vi "CAN Log Queue FGV Create the Reference.vi"(8 "error in":errorcluster, 11 "Selected Sockets":i16[](array[numeric])) -> (0 "error out":errorcluster)   [LabVIEW 2023, in "LTT_TeststandSteptypes.lvlib"]
uses:
  LTT_TeststandSteptypes.lvlib
  Control/CAN FGV State.ctl
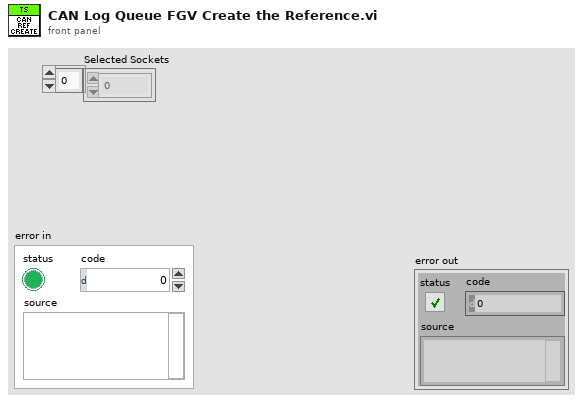
[diagram p1: front panel]
types:
  T1 = typedef "LTT_TeststandSteptypes.lvlib/CAN FGV State.ctl" = enum16{"Init", "Get", "Set"}
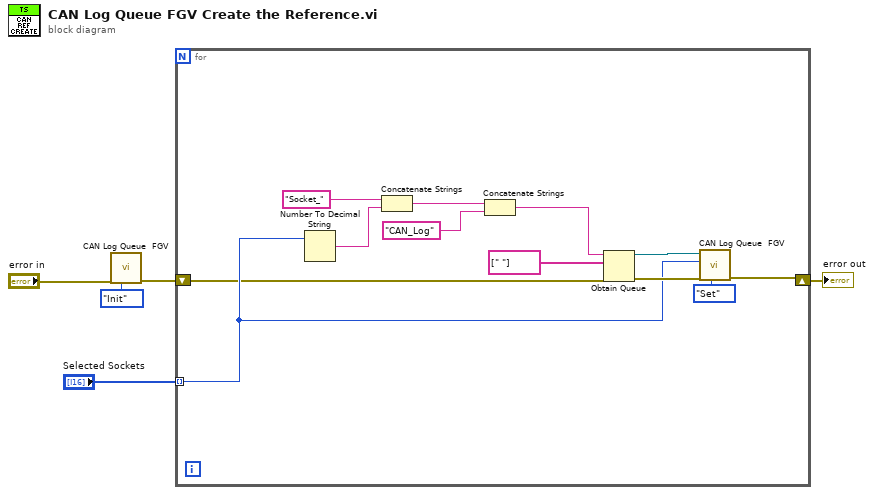
[diagram p0: block diagram]
diagram:
  n1 = call "CAN Log Queue  FGV.vi"("CAN FGV State"=CAN_FGV_State."Init", "error in"="error in") -> ("error out"=w2:errorcluster)  [unwired: 8 in, 1 out]
  n2 = for {
    tunnel: "Selected Sockets" -> [w7] mode=indexing
    shift-right: [w8] -> w1
    shift-left: w2 -> [w6]
    n3 = Number To Decimal String(number=w7) -> (decimal integer string=w16:string)  [unwired: 1 in]
    n4 = Concatenate Strings("Socket_" ("name (unnamed)"), w16) -> (w15:string)
    n5 = Concatenate Strings(w15, "CAN_Log" ("string")) -> (w14:string)
    n6 = Obtain Queue(name (unnamed)=w14, element data type=string[] [" "] ("appended array"), error in (no error)=w6) -> (queue out=w11:refnum<queue>, error out=w10:errorcluster)  [unwired: 2 in, 1 out]
    n7 = call "CAN Log Queue  FGV.vi"("CAN FGV State"=CAN_FGV_State."Set", "error in"=w10, "Current Scoket"=w7, "Log queue in"=w11) -> ("error out"=w8:errorcluster)  [unwired: 6 in, 1 out]
  }
  "error out" <- w1
